vi "MultiCombo.vi"(9 "String":string, 10 "Numeric":i32, 11 "Boolean":bool=TRUE) -> (1 "revString":string, 2 "String":string)   [LabVIEW 2020]
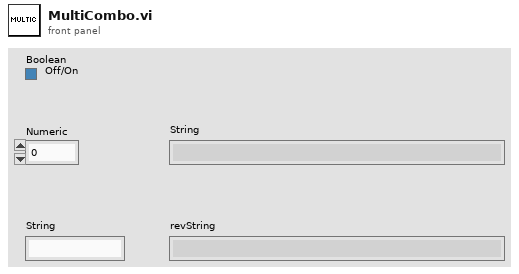
[diagram p1: front panel]
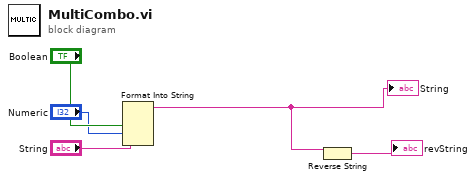
[diagram p0: block diagram]
diagram:
  n1 = Format Into String("Boolean", "Numeric", "String") -> (resulting string=w1:string)  [unwired: 3 in, 1 out]
  "String" <- w1
  n2 = Reverse String(1:w1) -> (0:→"revString":string)
